vi "To String.vi"(6 "pretty print? (T)":bool=TRUE, 7 "enable LabVIEW extensions? (T)":bool=TRUE, 8 "error in (no error)":errorcluster, 11 "JSON Value in":refnum<class "JSON Value.lvclass">) -> (0 "error out":errorcluster, 3 "String":string)   [LabVIEW 2016, in "JSON Value.lvclass"]
uses:
  JSON Value.lvclass
  JSON Value.lvclass/JSON Value.ctl
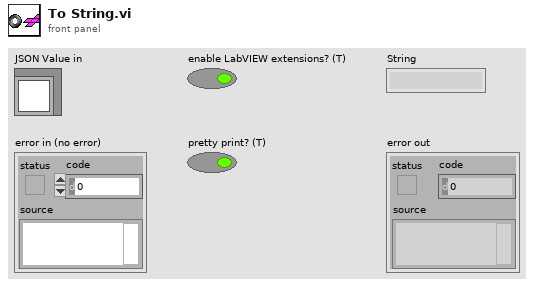
[diagram p1: front panel]
types:
  T1 = typedef "JSON Value.lvclass/JSON Types.ctl" = enum16{"String", "Numeric", "Boolean", "NULL", "Object", "Array"}
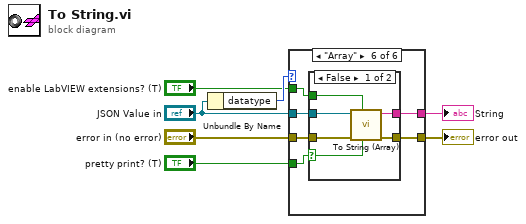
[diagram p0: block diagram]
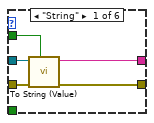
[diagram p2: hidden frame]
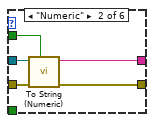
[diagram p3: hidden frame]
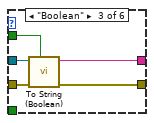
[diagram p4: hidden frame]
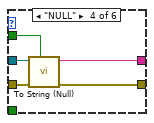
[diagram p5: hidden frame]
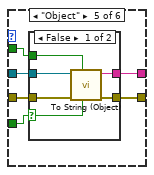
[diagram p6: hidden frame]
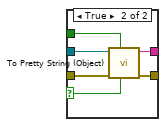
[diagram p7: hidden frame]
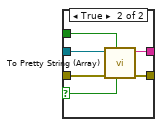
[diagram p8: hidden frame]
diagram:
  n1 = Unbundle By Name("JSON Value in") -> ("datatype"=w7:T1)
  n2 = case shown="\"Array\"" w7 {
    tunnel: [w12 w17 w22 w27 w33 w51] -> w6
    tunnel: [w11 w16 w21 w26 w32 w50] -> w5
    tunnel: "enable LabVIEW extensions? (T)" -> [w10 w15 w20 w25 w31 w49]
    tunnel: "error in (no error)" -> [w9 w14 w19 w24 w30 w48]
    tunnel: "JSON Value in" -> [w8 w13 w18 w23 w29 w47]
    tunnel: "pretty print? (T)" -> [_ _ _ _ w28 w46]
    frame "String" {
      n3 = call "To String (Value).vi"("enable LabVIEW extensions? (T)"=w10, "error in (no error)"=w9, "JSON Value in"=w8) -> ("error out"=w12:errorcluster, "String"=w11:string)  [unwired: 7 in]
    }
    frame "Numeric" {
      n4 = call "To String (Numeric).vi"("enable LabVIEW extensions? (T)"=w15, "error in (no error)"=w14, "JSON Value in"=w13) -> ("error out"=w17:errorcluster, "String"=w16:string)  [unwired: 7 in]
    }
    frame "Boolean" {
      n5 = call "To String (Boolean).vi"("enable LabVIEW extensions? (T)"=w20, "error in (no error)"=w19, "JSON Value in"=w18) -> ("error out"=w22:errorcluster, "String"=w21:string)  [unwired: 7 in]
    }
    frame "NULL" {
      n6 = call "To String (Null).vi"("enable LabVIEW extensions? (T)"=w25, "error in (no error)"=w24, "JSON Datatype in"=w23) -> ("error out"=w27:errorcluster, "String"=w26:string)  [unwired: 7 in]
    }
    frame "Object" {
      n7 = case shown="False" w28 {
        selector: w28 -> [w34 w45]
        tunnel: [w39 w41] -> w33
        tunnel: [w38 w43] -> w32
        tunnel: w31 -> [w37 w42]
        tunnel: w30 -> [w36 w40]
        tunnel: w29 -> [w35 w44]
        frame False {
          n8 = call "To String (Object).vi"("pretty print? (T)"=w34, "enable LabVIEW extensions? (T)"=w37, "error in (no error)"=w36, "JSON Value in"=w35) -> ("error out"=w39:errorcluster, "String"=w38:string)  [unwired: 6 in]
        }
        frame True {
          n9 = call "To Pretty String (Object).vi"("pretty print? (T)"=w45, "enable LabVIEW extensions? (T)"=w42, "error in (no error)"=w40, "JSON Value in"=w44) -> ("error out"=w41:errorcluster, "Pretty Print String"=w43:string)  [unwired: 6 in]
        }
      }
    }
    frame "Array" {
      n10 = case shown="False" w46 {
        selector: w46 -> [w52 w58]
        tunnel: [w57 w62] -> w51
        tunnel: [w56 w63] -> w50
        tunnel: w49 -> [w55 w59]
        tunnel: w48 -> [w54 w61]
        tunnel: w47 -> [w53 w60]
        frame False {
          n11 = call "To String (Array).vi"("pretty print? (T)"=w52, "enable LabVIEW extensions? (T)"=w55, "error in (no error)"=w54, "JSON Value in"=w53) -> ("error out"=w57:errorcluster, "String"=w56:string)  [unwired: 6 in]
        }
        frame True {
          n12 = call "To Pretty String (Array).vi"("pretty print? (T)"=w58, "enable LabVIEW extensions? (T)"=w59, "error in (no error)"=w61, "JSON Value in"=w60) -> ("error out"=w62:errorcluster, "Pretty Print String"=w63:string)  [unwired: 6 in]
        }
      }
    }
  }
  "error out" <- w6
  "String" <- w5
